vi "On New Image Available.vi"(8 "error in (no error)":errorcluster, 11 "ImageListener in":refnum<class "ImageListener.lvclass">) -> (0 "error out":errorcluster, 3 "ImageListener out":refnum<class "ImageListener.lvclass">)   [LabVIEW 2020, in "ImageListener.lvclass"]
uses:
  ImageListener.lvclass
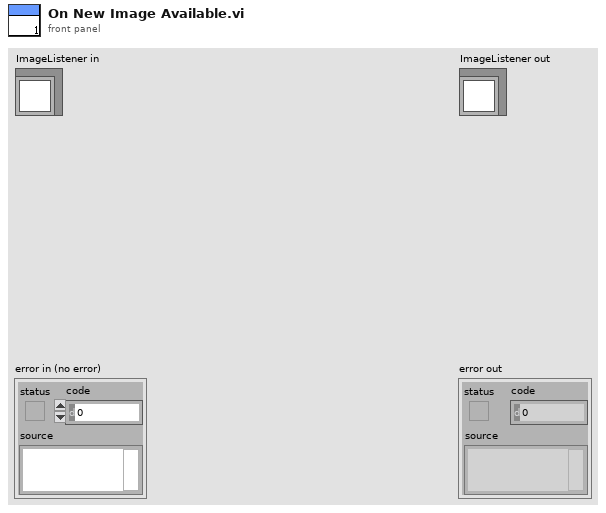
[diagram p1: front panel]
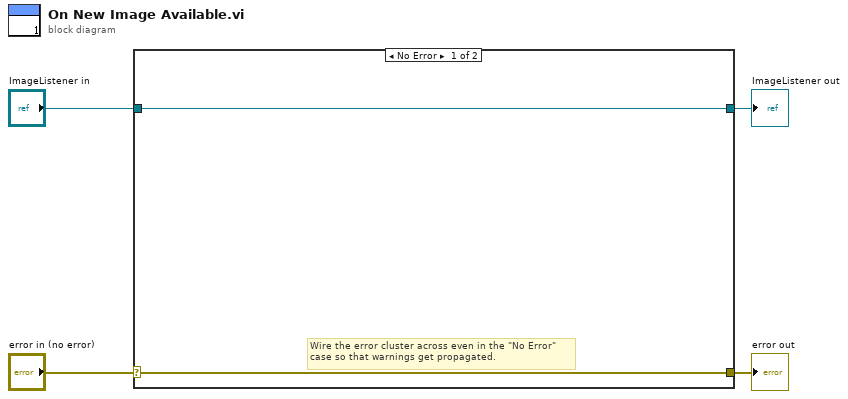
[diagram p0: block diagram]
diagram:
  n1 = case shown="No Error" "error in (no error)" {
    selector: "error in (no error)" -> [w5 w8]
    tunnel: [w5 w8] -> w3
    tunnel: [w6 w7] -> w1
    tunnel: "ImageListener in" -> [w6 w7]
    frame No Error {
      # "Wire the error cluster across even in the \"No Error\"\ncase so that warnings get propagated."
    }
    frame Error {
    }
  }
  "error out" <- w3
  "ImageListener out" <- w1
